vi "DAQmx.Acquire Recovery.vi"(8 "error in (no error)":errorcluster, 11 "DAQmx in":refnum<class "DAQmx.lvclass">) -> (0 "error out":errorcluster, 3 "DAQmx out":refnum<class "DAQmx.lvclass">)   [LabVIEW 2019, in "DAQmx.lvclass"]
uses:
  DAQmx.lvclass
  DAQmx.lvclass/DAQmx.ctl
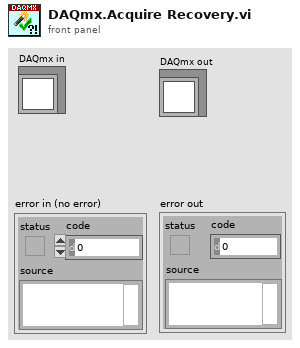
[diagram p1: front panel]
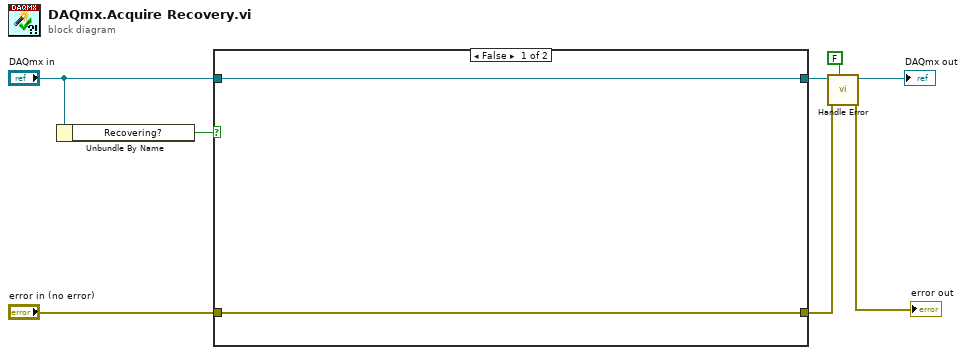
[diagram p0: block diagram]
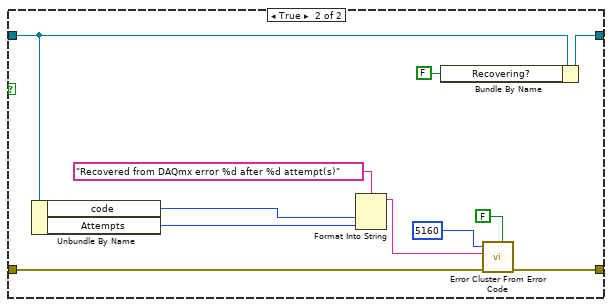
[diagram p2: hidden frame]
diagram:
  n1 = Unbundle By Name("DAQmx in") -> ("Recovering?"=w8:bool)
  n2 = case shown="False" w8 {
    tunnel: [w10 w12] -> w4
    tunnel: "DAQmx in" -> [w10 w11]
    tunnel: [w9 w16] -> w2
    tunnel: "error in (no error)" -> [w9 w15]
    frame False {
    }
    frame True {
      n3 = Unbundle By Name(w11) -> ("code"=w17:i32, "Attempts"=w18:i32)
      n4 = Format Into String(format string="Recovered from DAQmx error %d after %d attempt(s)", w17, w18) -> (resulting string=w19:string)  [unwired: 2 in, 1 out]
      n5 = Bundle By Name(cluster=w11, "Recovering?"=FALSE ("Recovery.Recovering?")) -> (w12:refnum<class "DAQmx.lvclass">)
      n6 = call <vilib>:"Error Cluster From Error Code.vi"("is warning? (False)"=FALSE, "error in (no error)"=w15, "error message (\"\")"=w19, "error code (0)"=5160 ("code")) -> ("error out"=w16:errorcluster)  [unwired: 5 in]
    }
  }
  n7 = call-dynamic "Handle Error.vi"("Stop on Unhandled Error (T)"=FALSE, "error in"=w2, "DAQmx"=w4) -> ("handling error"=→"error out":errorcluster, "DAQmx out"=→"DAQmx out":refnum<class "DAQmx.lvclass">)  [unwired: 6 in, 1 out]
